vi "Get Actual Button References.vi"(7 "Enum":T1, 8 "error in (no error)":errorcluster, 11 "\"Tab Forward To\" Refnum":refnum<vi>) -> (0 "error out":errorcluster, 3 "Refnum out":refnum<vi>)   [LabVIEW 2014, in "DCAFConfigurablePluginDecideFeatures.lvclass"]
uses:
  DCAFConfigurablePluginDecideFeatures.lvclass
  Button Names.ctl
  <vilib>/Utility/error.llb/Error Cluster From Error Code.vi
  <vilib>/ErrorRing/Error Ring.xnode
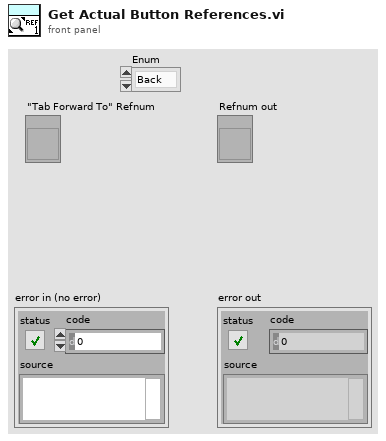
[diagram p1: front panel]
types:
  T1 = typedef "Button Names.ctl" = enum16{"Back", "Next", "Help", "Cancel"}
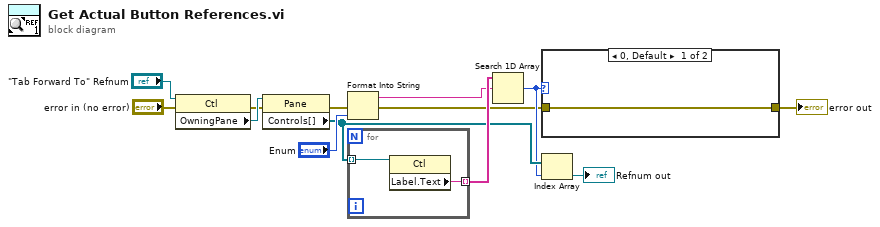
[diagram p0: block diagram]
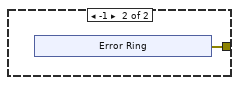
[diagram p2: hidden frame]
diagram:
  n1 = property class="Ctl"(reference="\"Tab Forward To\" Refnum", error in="error in (no error)") -> (error out=w11:errorcluster, "OwningPane"=w12:refnum<vi>)  [unwired: 1 out]
  n2 = property class="Pane"(reference=w12, error in=w11) -> (error out=w4:errorcluster, "Controls[]"=w6:refnum<vi>[])  [unwired: 1 out]
  n3 = Format Into String(error in=w4, "Enum") -> (resulting string=w7:string, error out=w1:errorcluster)  [unwired: 2 in]
  n4 = for {
    tunnel: w6 -> [w15] mode=indexing
    tunnel: [w14] -> w9 mode=indexing
    n5 = property class="Ctl"(reference=w15) -> ("Label.Text"=w14:string)  [unwired: 1 in, 2 out]
  }
  n6 = Search 1D Array(1D array=w9, element=w7) -> (index of element=w3:i32)  [unwired: 1 in]
  n7 = case shown="0, Default" w3 {
    tunnel: [w16 w17] -> w2
    tunnel: w1 -> [w16 _]
    frame 0, Default {
    }
    frame -1 {
      n8 = xnode "Error Ring"() -> ("error out"=w17:errorcluster)
    }
  }
  "error out" <- w2
  n9 = Index Array(array=w6, index=w3) -> (element=→"Refnum out":refnum<vi>)
